vi "DAQNavi Read (Analog 1D Wfm NChan 1Samp).vi"(8 "error in (no error)":errorcluster, 10 "timeout":dbl=10.0 format="%0.2f", 11 "task in":i32) -> (0 "error out":errorcluster, 2 "data":waveform(dbl)[](array[waveform]), 3 "task out":i32)   [LabVIEW 2020]
uses:
  DAQNavi_LV.dll
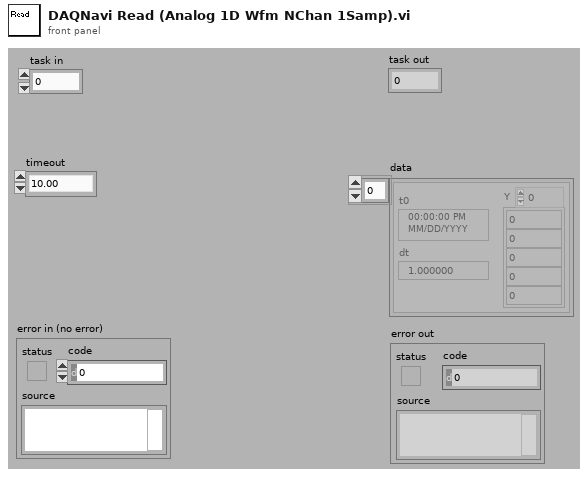
[diagram p1: front panel]
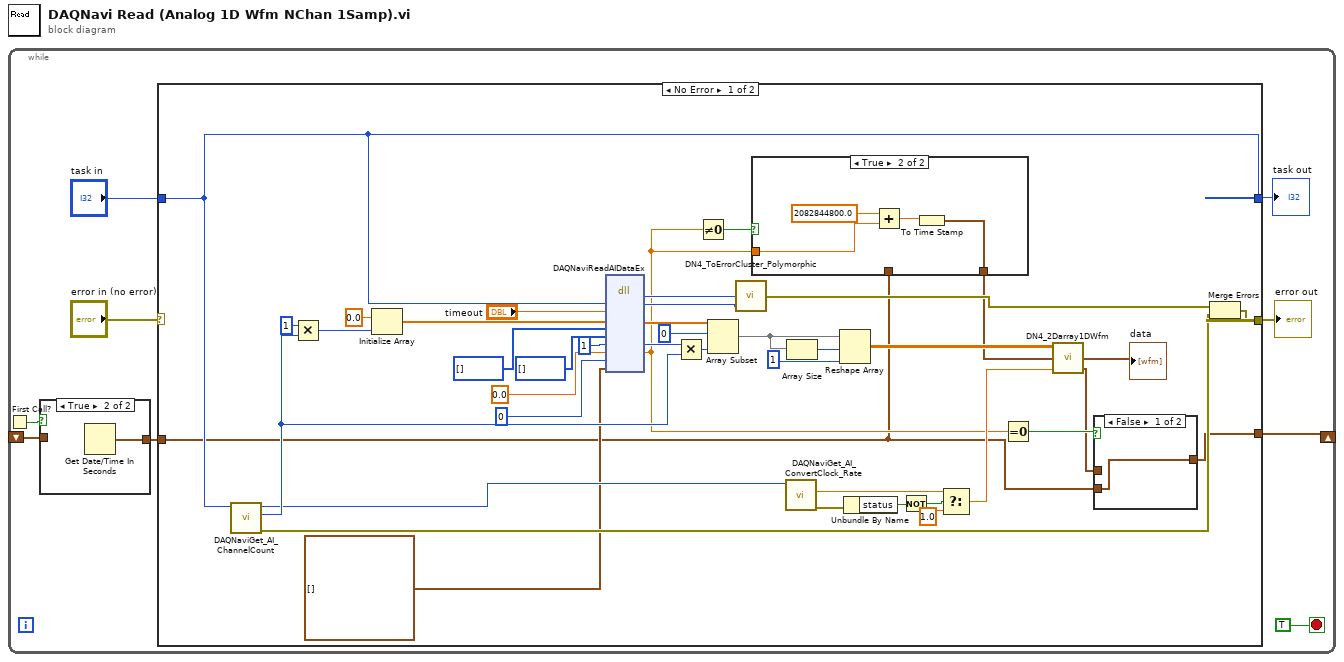
[diagram p0: block diagram]
diagram:
  n1 = while {
    shift-right: [w1] -> _
    shift-left: _ -> [w3]
    stop <- TRUE stop-if-true
    n2 = First Call?() -> (First Call?: T/F=w4:bool)
    n3 = case shown="True" w4 {
      tunnel: w3 -> [w10 _]
      tunnel: [w10 w11] -> w2
      frame False {
      }
      frame True {
        n4 = Get Date/Time In Seconds() -> (seconds since 1Jan1904=w11:timestamp)
      }
    }
    n5 = case shown="No Error" "error in (no error)" {
      selector: "error in (no error)" -> [_ w61]
      tunnel: "task in" -> [w22 w62]
      tunnel: [w22 w62] -> w7
      tunnel: [w43 w61] -> w6
      tunnel: w2 -> [w12 w60]
      tunnel: [w18 w60] -> w1
      frame No Error {
        n6 = call "DAQNaviGet_AI_ChannelCount.vi"("task in"=w22) -> ("error out"=w44:errorcluster, "channel count"=w37:i32, "task out"=w31:i32)  [unwired: 1 in, 7 out]
        n7 = Multiply(x=1 ("y"), y=w37) -> (x*y=w46:i32)
        n8 = Initialize Array(0.0 ("element"), w46) -> (w40:dbl[])
        n9 = dll-call lib="DAQNavi_LV.dll" fn="DAQNaviReadAIDataEx"("taskID"=w22, "timeout"="timeout", "scaledData"=w40, "rawData16"=u16[] [] ("scaledData"), "rawData32"=u32[] [], "samples"=u32 1, "startTime"=0.0, "markCount"=0 ("startTime"), "markBuf"=cluster{"DataIndex":i64, "SrcId":i64}[] []) -> ("return type"=w48:i32, "taskID"=w23:i32, "scaledData"=w39:dbl[], "samples"=w38:u32, "startTime"=w14:dbl)  [unwired: 4 in, 6 out]
        n10 = Multiply(x=w38, y=w37) -> (x*y=w36:u32)
        n11 = Not Equal To 0?(x=w14) -> (x != 0?=w15:bool)
        n12 = Array Subset(array=w39, index=0, length=w36) -> (w34:dbl[])
        n13 = call "DN4_ToErrorCluster_Polymorphic.vi"("task id"=w23, "error code"=w48) -> ("error out"=w45:errorcluster)  [unwired: 3 out]
        n14 = case shown="True" w15 {
          tunnel: w14 -> [_ w59]
          tunnel: [w55 w56] -> w13
          tunnel: w12 -> [w55 _]
          frame False {
          }
          frame True {
            n15 = Add(x=2082844800.0, y=w59) -> (x+y=w57:dbl)
            n16 = To Time Stamp(1:w57) -> (0:w56:timestamp)
          }
        }
        n17 = call "DAQNaviGet_AI_ConvertClock_Rate.vi"("task in"=w31) -> ("error out"=w30:errorcluster, "rate"=w27:dbl)  [unwired: 1 in, 8 out]
        n18 = Array Size(array=w34) -> (size(s)=w35:i32)
        n19 = Reshape Array(w34, w35, 1 ("dimension size")) -> (w32:dbl[][])
        n20 = Unbundle By Name(w30) -> ("status"=w29:bool)
        n21 = Not(x=w29) -> (.not. x?=w28:bool)
        n22 = Select(t=w27, s=w28, f=1.0) -> (s? t:f=w25:dbl)
        n23 = Equal To 0?(x=w14) -> (x = 0?=w20:bool)
        n24 = call "DN4_2Darray1DWfm.vi"("rate"=w25, "StartTime"=w13, "2D Array"=w32) -> ("EndTime"=w19:timestamp, "1D Wfm"=→"data":waveform(dbl)[])  [unwired: 1 in]
        n25 = case shown="False" w20 {
          tunnel: w19 -> [_ w54]
          tunnel: w12 -> [w53 _]
          tunnel: [w53 w54] -> w18
          frame False {
          }
          frame True {
          }
        }
        n26 = Merge Errors(w45, w44) -> (w43:errorcluster)
      }
      frame Error {
      }
    }
    "task out" <- w7
    "error out" <- w6
  }
